vi "Write Cluster.vi"(8 "error in (no error)":errorcluster, 10 "Cluster":T1, 11 "CallRequest (JSON) in":refnum<class "CallRequest (JSON).lvclass">) -> (0 "error out":errorcluster, 3 "CallRequest (JSON) out":refnum<class "CallRequest (JSON).lvclass">)   [LabVIEW 2020, in "wamplv.lvlib" / "CallRequest (JSON).lvclass"]
uses:
  CallRequest (JSON).lvclass
  TypeDefs/CALL request (JSON).ctl
  WAMP Client/API/TypeDefs/RESULT payload (JSON).ctl
  WAMP Client/API/TypeDefs/Combined error.ctl
  WAMP Client/API/TypeDefs/WAMP error.ctl
  CallRequest (JSON).lvclass/CallRequest (JSON).ctl
  WAMP Client/WAMP Client.lvclass
  wamplv.lvlib
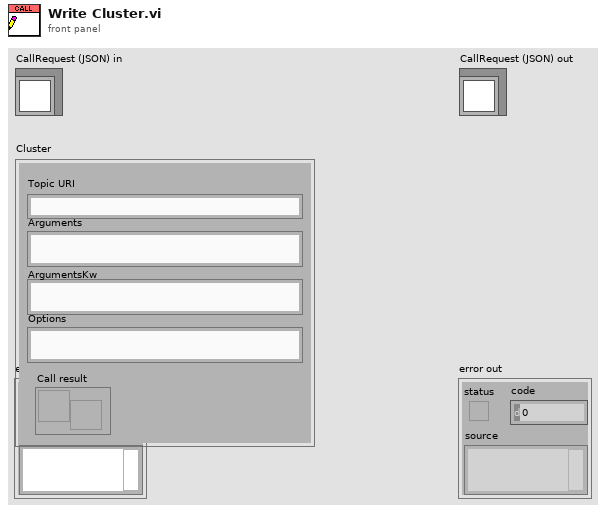
[diagram p1: front panel]
types:
  T1 = typedef "wamplv.lvlib/CALL request (JSON).ctl" = cluster{"Topic URI":string, "Arguments":string, "ArgumentsKw":string, "Options":string, "Call result":refnum<notifier>}
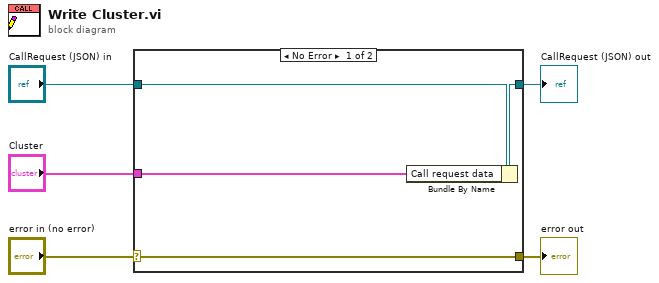
[diagram p0: block diagram]
diagram:
  n1 = case shown="No Error" "error in (no error)" {
    selector: "error in (no error)" -> [w9 w10]
    tunnel: [w9 w10] -> w4
    tunnel: [w7 w11] -> w2
    tunnel: "CallRequest (JSON) in" -> [w8 w11]
    tunnel: "Cluster" -> [w6 _]
    frame No Error {
      n2 = Bundle By Name(cluster=w8, "Call request data"=w6) -> (w7:refnum<class "CallRequest (JSON).lvclass">)
    }
    frame Error {
    }
  }
  "error out" <- w4
  "CallRequest (JSON) out" <- w2
